vi "matlab_write.vi"(4 "error in":errorcluster, 5 "data in":variant, 6 "name":string, 7 "ref in":T1 format="%.0x") -> (0 "error out":errorcluster, 3 "ref out":T1 format="%.0x")   [LabVIEW 2019]
uses:
  <vilib>/addons/h5labview2/base/hid_t.ctl
  <vilib>/addons/h5labview2/base/lib_path.vi
  <vilib>/addons/h5labview2/base/H5Equery.vi
  <vilib>/addons/h5labview2/attrib/H5Awrite.llb/H5Awrite.xnode
  <vilib>/addons/h5labview2/group/H5G.lvlib
  <vilib>/addons/h5labview2/dataset/H5D.lvlib
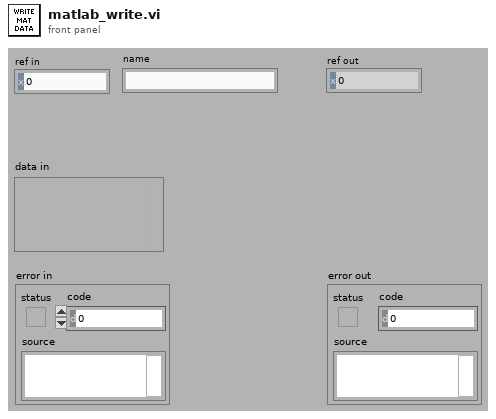
[diagram p1: front panel]
types:
  T1 = typedef "hid_t.ctl" = i32
  T2 = typedef "Type Descriptor Enumeration__ogtk.ctl" = enum8{"<Null>", "I8", "I16", "I32", "I64", "U8", "U16", "U32", "U64", "SGL", "DBL", "EXT", "CSG", "CDB", "CXT", "0x0F", "0x10", "0x11", "0x12", "0x13", "0x14", "Enum U8", "Enum U16", "Enum U32", "Enum U64", "SGL PQ", "DBL PQ", "EXT PQ", "CSG PQ", "CDB PQ", "CXT PQ", "0x1F", "0x20", "Boolean", "0x22", "0x23", "0x24", "0x25", "0x26", "0x27", "0x28", "0x29", "0x2A", "0x2B", "0x2C", "0x2D", "0x2E", "0x2F", "String", "0x31", "Path", "Pict", "0x34", "0x35", "0x36", "DAQ", "0x38", "0x39", "0x3A", "0x3B", "0x3C", "0x3D", "0x3E", "0x3F", "Array", "0x41", "0x42", "0x43", "0x44", "0x45", "0x46", "0x47", "0x48", "0x49", "0x4A", "0x4B", "0x4C", "0x4D", "0x4E", "0x4F", "Cluster", "0x51", "0x52", "Variant", "Waveform", "0x55", "0x56", "0x57", "0x58", "0x59", "0x5A", "0x5B", "0x5C", "0x5D", "0x5E", "0x5F", "0x60", "0x61", "0x62", "0x63", "0x64", "0x65", "0x66", "0x67", "0x68", "0x69", "0x6A", "0x6B", "0x6C", "0x6D", "0x6E", "0x6F", "Refnum"}
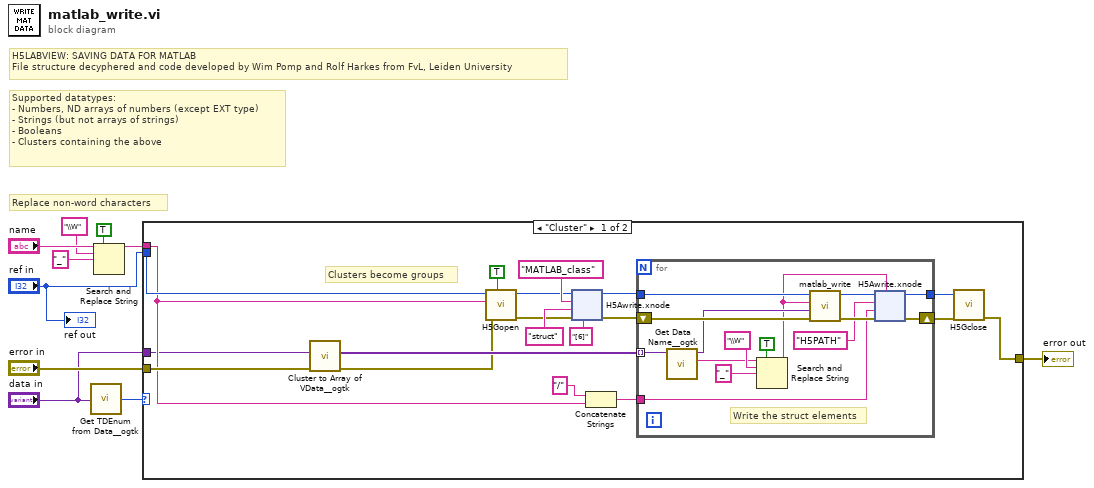
[diagram p0: block diagram]
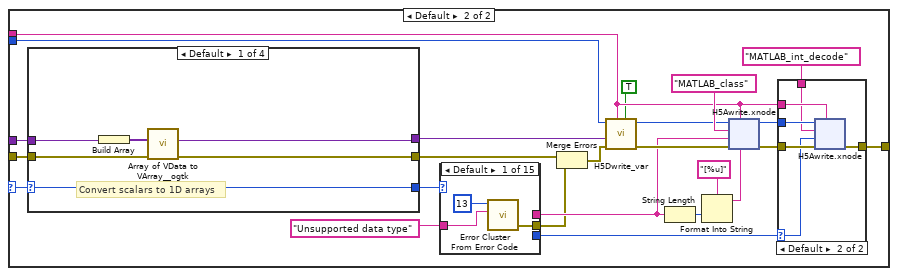
[diagram p2: hidden frame]
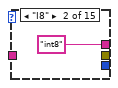
[diagram p4: hidden frame]
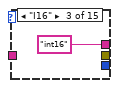
[diagram p5: hidden frame]
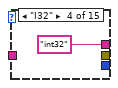
[diagram p6: hidden frame]
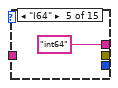
[diagram p7: hidden frame]
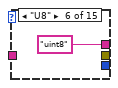
[diagram p8: hidden frame]
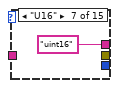
[diagram p9: hidden frame]
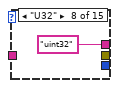
[diagram p10: hidden frame]
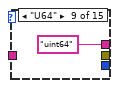
[diagram p11: hidden frame]
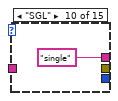
[diagram p12: hidden frame]
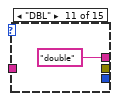
[diagram p13: hidden frame]
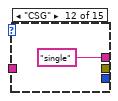
[diagram p14: hidden frame]
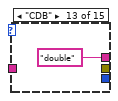
[diagram p15: hidden frame]
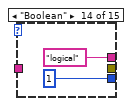
[diagram p16: hidden frame]
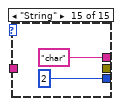
[diagram p17: hidden frame]
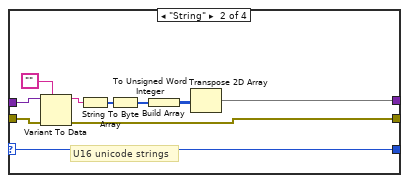
[diagram p18: hidden frame]
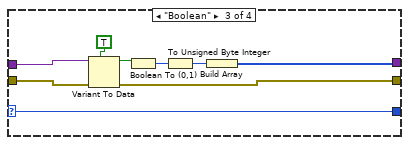
[diagram p19: hidden frame]
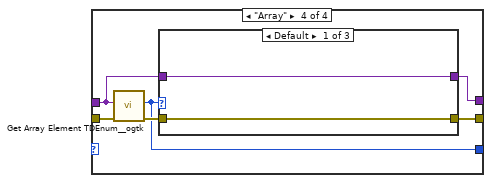
[diagram p20: hidden frame]
diagram:
  # "Supported datatypes:\n- Numbers, ND arrays of numbers (except EXT type)\n- Strings (but not arrays of strings)\n- Booleans\n- Clusters containing the above"
  # "H5LABVIEW: SAVING DATA FOR MATLAB\nFile structure decyphered and code developed by Wim Pomp and Rolf Harkes from FvL, Leiden University"
  # "Replace non-word characters"
  n1 = call <userlib>:"Get TDEnum from Data__ogtk.vi"("Data"="data in") -> ("Type Descriptor Enumeration"=w9:T2)  [unwired: 4 in]
  n2 = Search and Replace String(replace all?=TRUE ("replace all? (F)"), input string="name", search string="\\W", replace string="_" ("replace string (\"\")")) -> (result string=w7:string)  [unwired: 4 in, 3 out]
  n3 = case shown="\"Cluster\"" w9 {
    selector: w9 -> [_ w100]
    tunnel: "error in" -> [w29 w102]
    tunnel: "data in" -> [w12 w85]
    tunnel: w7 -> [w15 w95]
    tunnel: "ref in" -> [w20 w92]
    tunnel: [w21 w91] -> w8
    frame "Cluster" {
      # "Clusters become groups"
      n4 = call <userlib>:"Cluster to Array of VData__ogtk.vi"("error in (no error)"=w29, "Cluster"=w12) -> ("error out"=w19:errorcluster, "Array of VData"=w25:variant[])  [unwired: 8 in]
      n5 = call <vilib>:"H5Gopen.vi"("create? (F)"=TRUE, "error in (no error)"=w19, "name"=w15, "ref in"=w20) -> ("error out"=w18:errorcluster, "group out"=w17:T1)  [unwired: 6 in]
      n6 = xnode "H5Awrite.xnode"("type name (default)"="[6]", "error in (no error)"=w18, "data"="struct" ("attrib name"), "attrib name"="MATLAB_class", "ref in"=w17) -> ("error out"=w23:errorcluster, "ref out"=w24:i32)  [unwired: 2 in, 1 out]
      n7 = Concatenate Strings("/", w15) -> (w14:string)
      n8 = for {
        tunnel: w25 -> [w42] mode=indexing
        tunnel: w24 -> [w41]
        shift-right: [w37] -> w22
        shift-left: w23 -> [w40]
        tunnel: [w38] -> w16
        tunnel: w14 -> [w35]
        # "Write the struct elements"
        n9 = call <userlib>:"Get Data Name__ogtk.vi"("Data"=w42) -> ("Data Name"=w31:string, "Data dup"=w39:variant)  [unwired: 8 in, 1 out]
        n10 = Search and Replace String(replace all?=TRUE ("replace all? (F)"), input string=w31, search string="\\W", replace string="_" ("replace string (\"\")")) -> (result string=w30:string)  [unwired: 4 in, 3 out]
        n11 = call "matlab_write.vi"("error in"=w40, "data in"=w39, "name"=w30, "ref in"=w41) -> ("error out"=w37:errorcluster, "ref out"=w38:T1)  [unwired: 2 in]
        n12 = xnode "H5Awrite.xnode"("object name"=w30, "error in (no error)"=w37, "data"=w35, "attrib name"="H5PATH", "ref in"=w38) -> ()  [unwired: 2 in, 3 out]
      }
      n13 = call <vilib>:"H5Gclose.vi"("error in (no error)"=w22, "group in"=w16) -> ("error out"=w21:errorcluster)  [unwired: 9 in]
    }
    frame Default {
      n14 = case shown="Default" w100 {
        selector: w100 -> [w170 w178 w187 _]
        tunnel: [w170 w178 w187 w191] -> w101
        tunnel: w102 -> [w166 w180 w189 w195]
        tunnel: [w165 w176 w186 w190] -> w81
        tunnel: w85 -> [w168 w179 w188 w194]
        tunnel: [w169 w173 w181 w193] -> w84
        frame Default {
          # "Convert scalars to 1D arrays"
          n15 = Build Array(w168) -> (w167:variant[])
          n16 = call <userlib>:"Array of VData to VArray__ogtk.vi"("error in (no error)"=w166, "1D Array of VData"=w167) -> ("error out"=w165:errorcluster, "VArray"=w169:variant)  [unwired: 8 in]
        }
        frame "String" {
          # "U16 unicode strings"
          n17 = Variant To Data(error in=w180, type="", Variant=w179) -> (data=w175:string, error out=w176:errorcluster)
          n18 = String To Byte Array(string=w175) -> (unsigned byte array=w174:u8[])
          n19 = To Unsigned Word Integer(number=w174) -> (unsigned 16bit integer=w172:u16[])
          n20 = Build Array(w172) -> (w171:u16[][])
          n21 = Transpose 2D Array(2D array=w171) -> (transposed array=w173:u16[][])
        }
        frame "Boolean" {
          n22 = Variant To Data(error in=w189, type=TRUE, Variant=w188) -> (data=w184:bool, error out=w186:errorcluster)
          n23 = Boolean To (0,1)(Boolean=w184) -> (0, 1=w183:i16)
          n24 = To Unsigned Byte Integer(number=w183) -> (unsigned 8bit integer=w182:u8)
          n25 = Build Array(w182) -> (w181:u8[])
        }
        frame "Array" {
          n26 = call <userlib>:"Get Array Element TDEnum__ogtk.vi"("error in (no error)"=w195, "Array"=w194) -> ("error out"=w192:errorcluster, "Element Type"=w191:T2)  [unwired: 8 in]
          n27 = case shown="Default" w191 {
            tunnel: w194 -> [w197 _ w205]
            tunnel: [w197 _ w204] -> w193
            tunnel: w192 -> [w196 w201 w203]
            tunnel: [w196 w200 w202] -> w190
            frame Default {
            }
            frame "String" {
              n28 = call <vilib>:"Error Cluster From Error Code.vi"("error in (no error)"=w201, "error message (\"\")"="Arrays of strings unsupported" ("search string"), "error code (0)"=13) -> ("error out"=w200:errorcluster)  [unwired: 6 in]
            }
            frame "Boolean" {
              # "Reinterp as U8"
              n29 = Variant To Flattened String(Variant=w205) -> (data string=w206:string, 1:w207:i16[])
              n30 = Index Array(array=w207, index=2) -> (element=w212:i16)
              n31 = expression code="2*x+4"(w212) -> (w208:i16)
              n32 = Replace Array Subset(array=w207, new element=i16 5 ("new element/subarray"), index=w208) -> (w209:i16[])
              n33 = Flattened String To Variant(4:w203, 6:w206, 7:w209) -> (0:w202:errorcluster, 3:w204:variant)
            }
          }
        }
      }
      n34 = case shown="Default" w101 {
        tunnel: [_ "int8" "int16" "int32" "int64" "uint8" "uint16" "uint32" "uint64" "single" "double" "single" "double" "logical" "char"] -> w89
        tunnel: [_ _ _ _ _ _ _ _ _ _ _ _ _ 1 2] -> w99
        tunnel: [w147 _ _ _ _ _ _ _ _ _ _ _ _ _ _] -> w82
        tunnel: "Unsupported data type" ("search string") -> [w146 _ _ _ _ _ _ _ _ _ _ _ _ _ _]
        frame Default {
          n35 = call <vilib>:"Error Cluster From Error Code.vi"("error message (\"\")"=w146, "error code (0)"=13) -> ("error out"=w147:errorcluster)  [unwired: 7 in]
        }
        frame "I8" {
        }
        frame "I16" {
        }
        frame "I32" {
        }
        frame "I64" {
        }
        frame "U8" {
        }
        frame "U16" {
        }
        frame "U32" {
        }
        frame "U64" {
        }
        frame "SGL" {
        }
        frame "DBL" {
        }
        frame "CSG" {
        }
        frame "CDB" {
        }
        frame "Boolean" {
        }
        frame "String" {
        }
      }
      n36 = Merge Errors(w81, w82) -> (w83:errorcluster)
      n37 = call <vilib>:"H5Dwrite_var.vi"("replace? (F)"=TRUE, "dataset name"=w95, "error in (no error)"=w83, "data"=w84, "ref in"=w92) -> ("error out"=w93:errorcluster, "ref out"=w94:T1)  [unwired: 4 in, 1 out]
      n38 = String Length(string=w89) -> (length=w88:i32)
      n39 = Format Into String(format string="[%u]", w88) -> (resulting string=w87:string)  [unwired: 2 in, 1 out]
      n40 = xnode "H5Awrite.xnode"("type name (default)"=w87, "object name"=w95, "error in (no error)"=w93, "data"=w89, "attrib name"="MATLAB_class", "ref in"=w94) -> ("error out"=w97:errorcluster, "ref out"=w98:T1)  [unwired: 1 in, 1 out]
      n41 = case shown="Default" w99 {
        selector: w99 -> [_ w125]
        tunnel: w98 -> [_ w127]
        tunnel: w97 -> [w121 w126]
        tunnel: [w121 w124] -> w91
        tunnel: w95 -> [_ w123]
        tunnel: "MATLAB_int_decode" ("attrib name") -> [_ w122]
        frame 0 {
        }
        frame Default {
          n42 = xnode "H5Awrite.xnode"("object name"=w123, "error in (no error)"=w126, "data"=w125, "attrib name"=w122, "ref in"=w127) -> ("error out"=w124:errorcluster)  [unwired: 2 in, 2 out]
        }
      }
    }
  }
  "error out" <- w8
  "ref out" <- "ref in"
